vi "Update Min Pass Number.vi"(8 "error in":errorcluster, 10 "Curr Cal Cfg":T1, 11 "Ctrl Ref":T2) -> (0 "error out":errorcluster, 2 "Curr Cal Cfg Out":T1)   [LabVIEW 2020, in "GUCalibration2.lvlib"]
uses:
  GUCalibration2.lvlib
  Controls/GU Arrange UI Ref.ctl
  Controls/Config Data Type.ctl
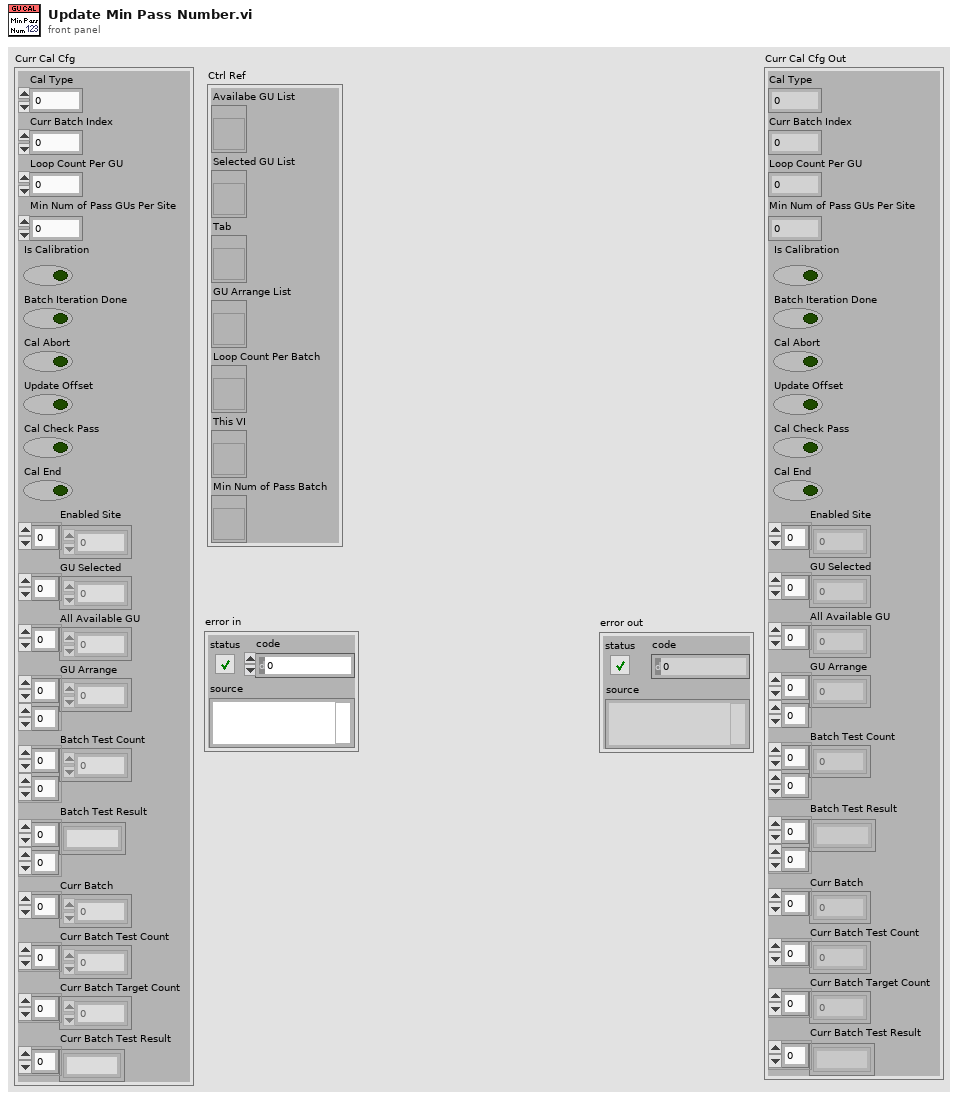
[diagram p1: front panel]
types:
  T1 = typedef "GUCalibration2.lvlib/Config Data Type.ctl" = cluster{"Cal Type":i32, "Curr Batch Index":i32, "Loop Count Per GU":i32, "Min Num of Pass GUs Per Site":i32, "Is Calibration":bool, "Batch Iteration Done":bool, "Cal Abort":bool, "Update Offset":bool, "Cal Check Pass":bool, "Cal End":bool, "Enabled Site":i32[], "GU Selected":i32[], "All Available GU":i32[], "GU Arrange":i32[][], "Batch Test Count":i32[][], "Batch Test Result":string[][], "Curr Batch":i32[], "Curr Batch Test Count":i32[], "Curr Batch Target Count":i32[], "Curr Batch Test Result":string[]}
  T2 = typedef "GUCalibration2.lvlib/GU Arrange UI Ref.ctl" = cluster{"Availabe GU List":refnum<vi>, "Selected GU List":refnum<vi>, "Tab":refnum<vi>, "GU Arrange List":refnum<vi>, "Loop Count Per Batch":refnum<vi>, "This VI":refnum<vi>, "Min Num of Pass Batch":refnum<vi>}
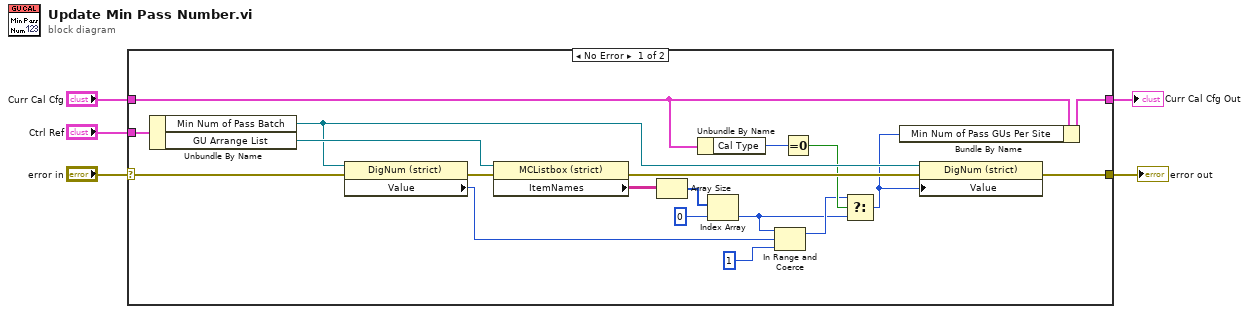
[diagram p0: block diagram]
diagram:
  n1 = case shown="No Error" "error in" {
    selector: "error in" -> [w15 w25]
    tunnel: "Ctrl Ref" -> [w19 _]
    tunnel: "Curr Cal Cfg" -> [w11 w26]
    tunnel: [w17 w25] -> w3
    tunnel: [w16 w26] -> w2
    frame No Error {
      n2 = Unbundle By Name(w19) -> ("Min Num of Pass Batch"=w13:refnum<vi>, "GU Arrange List"=w18:refnum<vi>)
      n3 = property on="Property Node" class="DigNum (strict)"(reference=w13, error in=w15) -> (error out=w14:errorcluster, "Value"=w12:i32)  [unwired: 1 out]
      n4 = property on="Property Node" class="MCListbox (strict)"(reference=w18, error in=w14) -> (error out=w23:errorcluster, "ItemNames"=w22:string[][])  [unwired: 1 out]
      n5 = Array Size(array=w22) -> (size(s)=w21:i32[])
      n6 = Unbundle By Name(w11) -> ("Cal Type"=w10:i32)
      n7 = Index Array(array=w21, index=0) -> (element=w7:i32)
      n8 = In Range and Coerce(upper limit=w7, x=w12, lower limit=1) -> (coerced(x)=w8:i32)  [unwired: 1 out]
      n9 = Equal To 0?(x=w10) -> (x = 0?=w9:bool)
      n10 = Select(t=w8, s=w9, f=w7) -> (s? t:f=w6:i32)
      n11 = Bundle By Name(cluster=w11, "Min Num of Pass GUs Per Site"=w6) -> (w16:T1)
      n12 = property on="Property Node" class="DigNum (strict)"(reference=w13, error in=w23, "Value"=w6) -> (error out=w17:errorcluster)  [unwired: 1 out]
    }
    frame Error {
    }
  }
  "error out" <- w3
  "Curr Cal Cfg Out" <- w2
